vi "Database Saver.vi"(11 "Command":string) -> ()   [LabVIEW 2023]
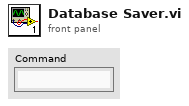
[diagram p1: front panel]
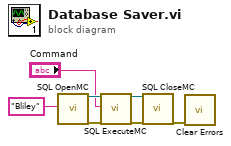
[diagram p0: block diagram]
diagram:
  n1 = call "SQL OpenMC.vi"("ConnectionString In"="Bliley") -> ("Connection Out"=w6:refnum<k7>, "Error out"=w5:errorcluster)  [unwired: 17 in]
  n2 = call "SQL ExecuteMC.vi"("Connection In"=w6, "SQL Query"="Command", "Error in (no error)"=w5) -> ("Connection Out"=w3:refnum<k7>, "Error out"=w4:errorcluster)  [unwired: 15 in]
  n3 = call "SQL CloseMC.vi"("Connection In"=w3, "Error in (no error)"=w4) -> ("Error out"=w2:errorcluster)  [unwired: 17 in]
  n4 = call <vilib>:"Clear Errors.vi"("error in (no error)"=w2) -> ()  [unwired: 5 in, 2 out]
